vi "Transform And Project Single Object.vi"(6 "Backface Culling Enabled":bool, 7 "Light Direction":T1={"x"=0.0, "y"=10.0, "z"=-10.0}, 8 "Object":T3 {"Triangles"."Vertex 3"."UV"."v" min=0 max=1 step=0.1; "Triangles"."Vertex 3"."UV"."u" min=0 max=1 step=0.1; "Triangles"."Vertex 2"."UV"."v" min=0 max=1 step=0.1; "Triangles"."Vertex 2"."UV"."u" min=0 max=1 step=0.1; "Triangles"."Vertex 1"."UV"."v" min=0 max=1 step=0.1; "Triangles"."Vertex 1"."UV"."u" min=0 max=1 step=0.1}, 9 "View Matrix":sgl[][](array[numeric]), 10 "Projection Matrix":sgl[][](array[numeric]), 11 "Screen Dimensions":T2) -> (3 "Triangles":T4[](array[typedef]) {"Vertex 3"."UV"."v" min=0 max=1 step=0.1; "Vertex 3"."UV"."u" min=0 max=1 step=0.1; "Vertex 2"."UV"."v" min=0 max=1 step=0.1; "Vertex 2"."UV"."u" min=0 max=1 step=0.1; "Vertex 1"."UV"."v" min=0 max=1 step=0.1; "Vertex 1"."UV"."u" min=0 max=1 step=0.1})   [LabVIEW 2020, in "Scene.lvclass"]
uses:
  Scene/Scene.lvclass
  Scene/Scene.lvclass/Scene.ctl
  Graphics/Libraries/3D/3D.lvlib
  Graphics/Libraries/3D/Vector 3D.ctl
  Graphics/Libraries/Raster/UV.ctl
  Graphics/Libraries/Raster/Raster.lvlib
  Graphics/Libraries/3D/Vertex.ctl
  Graphics/Libraries/3D/Triangle.ctl
  Graphics/Libraries/Raster/Rectangle Dimensions.ctl
  Graphics/Libraries/Raster/Texture.ctl
  Graphics/Libraries/3D/Material.ctl
  Graphics/Libraries/3D/Transform.ctl
  Graphics/Libraries/3D/Object.ctl
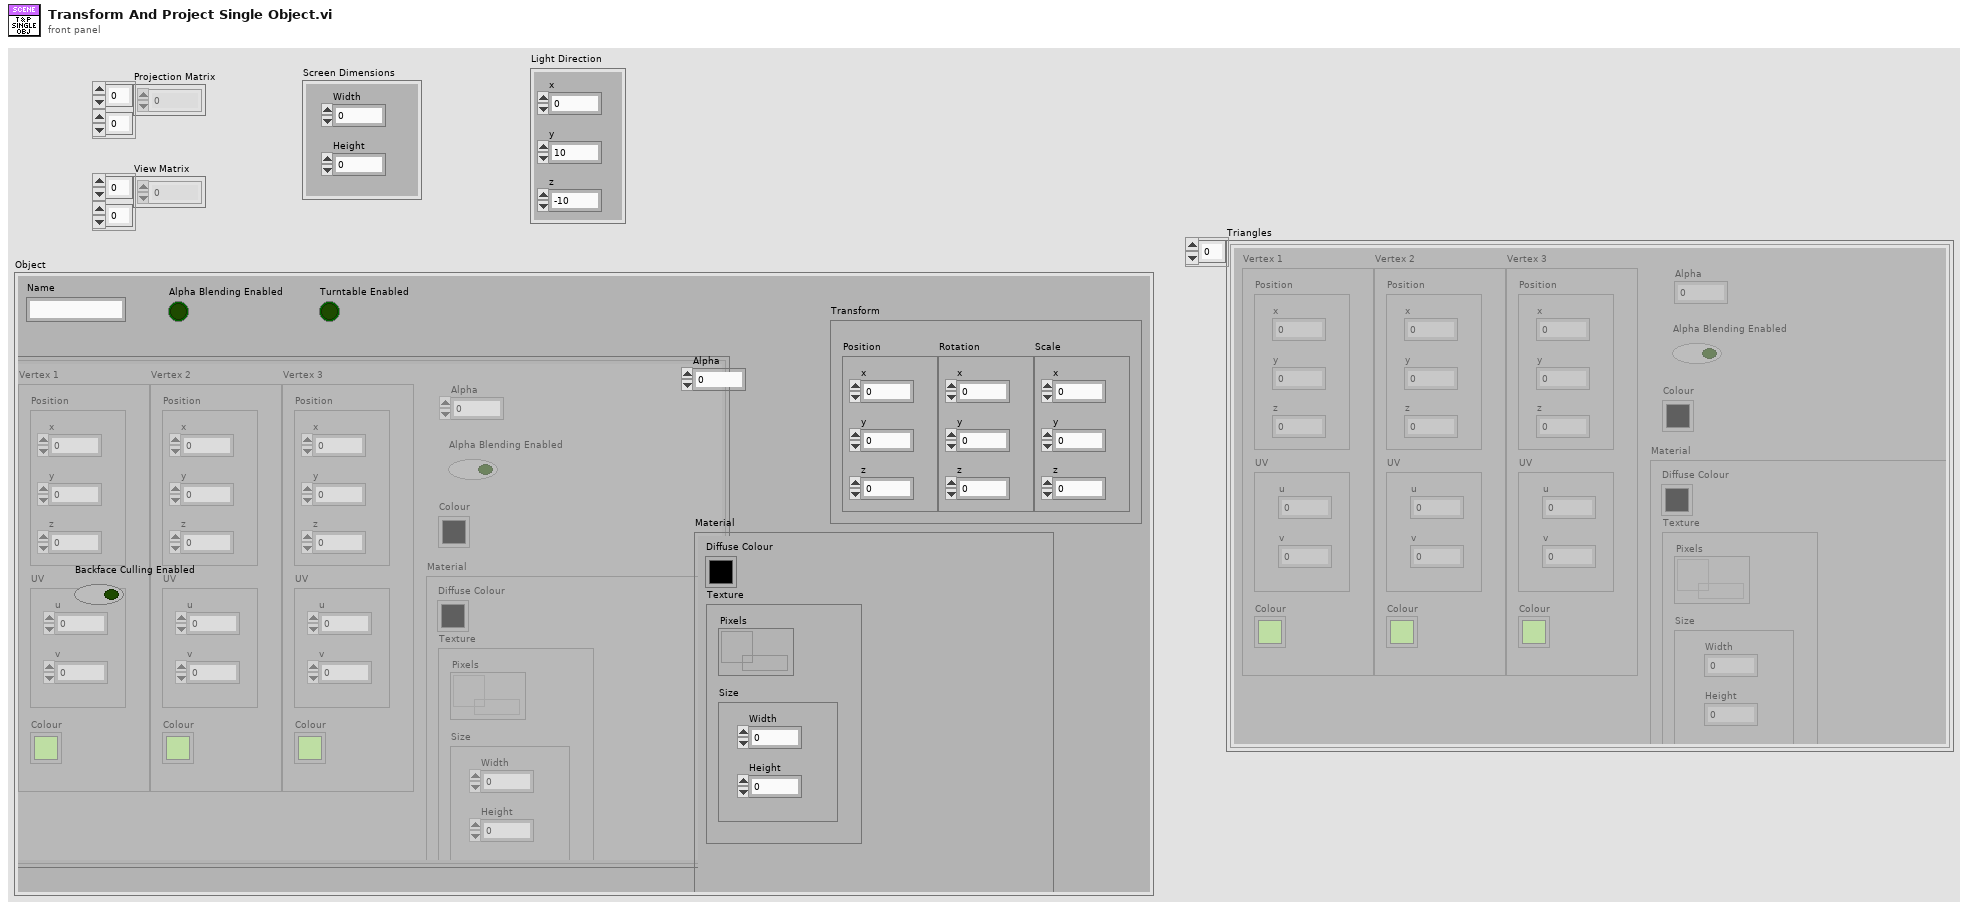
[diagram p1: front panel]
types:
  T1 = typedef "3D.lvlib/Vector 3D.ctl" = cluster{"x":sgl, "y":sgl, "z":sgl}
  T2 = typedef "Raster.lvlib/Rectangle Dimensions.ctl" = cluster{"Width":u32, "Height":u32}
  T3 = typedef "3D.lvlib/Object.ctl" = cluster{"Triangles":T4[], "Transform":T9, "Name":string, "Alpha Blending Enabled":bool, "Alpha":dbl, "Turntable Enabled":bool, "Material":T7}
  T4 = typedef "3D.lvlib/Triangle.ctl" = cluster{"Vertex 1":T5, "Vertex 2":T5, "Vertex 3":T5, "Alpha":dbl, "Alpha Blending Enabled":bool, "Colour":u32, "Material":T7}
  T5 = typedef "3D.lvlib/Vertex.ctl" = cluster{"Position":T1, "UV":T6, "Colour":u32}
  T6 = typedef "Raster.lvlib/UV.ctl" = cluster{"u":sgl, "v":sgl}
  T7 = typedef "3D.lvlib/Material.ctl" = cluster{"Diffuse Colour":u32, "Texture":T8}
  T8 = typedef "Raster.lvlib/Texture.ctl" = cluster{"Pixels":refnum<data-value>, "Size":T2}
  T9 = typedef "3D.lvlib/Transform.ctl" = cluster{"Position":T1, "Rotation":T1, "Scale":T1}
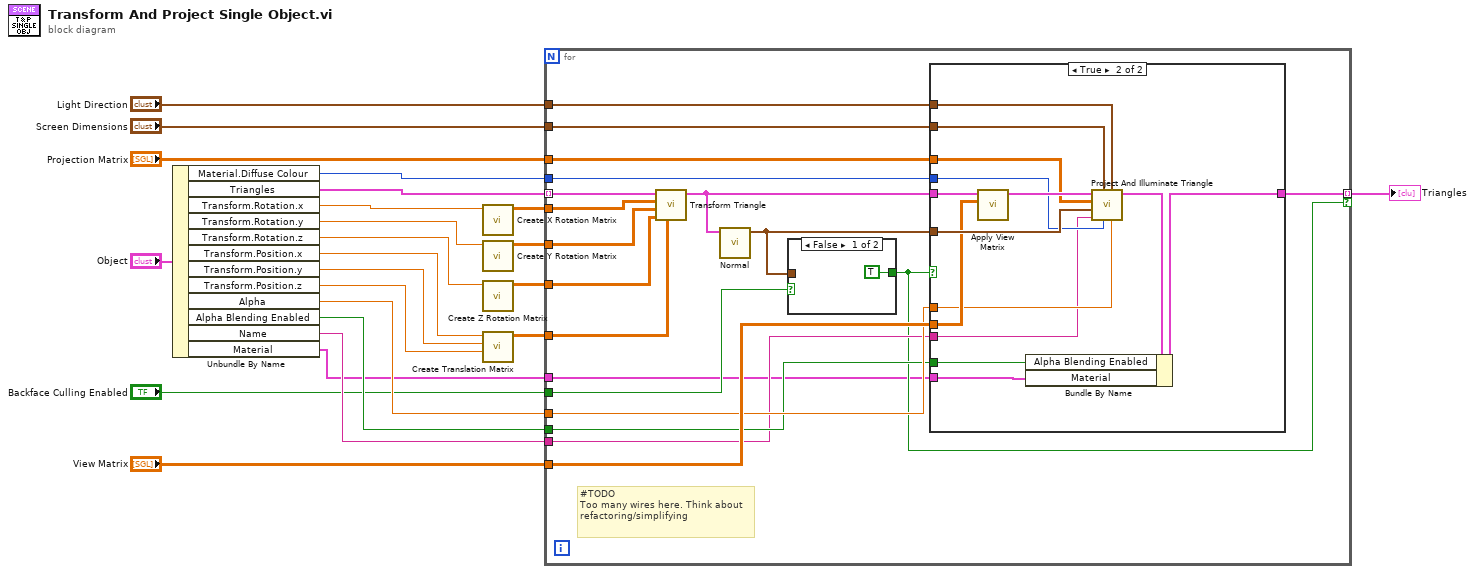
[diagram p0: block diagram]
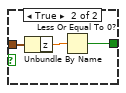
[diagram p2: hidden frame]
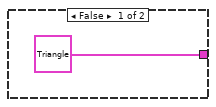
[diagram p3: hidden frame]
diagram:
  n1 = Unbundle By Name("Object") -> ("Material.Diffuse Colour"=w15:u32, "Triangles"=w8:T4[], "Transform.Rotation.x"=w16:sgl, "Transform.Rotation.y"=w17:sgl, "Transform.Rotation.z"=w18:sgl, "Transform.Position.x"=w19:sgl, "Transform.Position.y"=w20:sgl, "Transform.Position.z"=w21:sgl, "Alpha"=w22:dbl, "Alpha Blending Enabled"=w5:bool, "Name"=w3:string, "Material"=w1:T7)
  n2 = call "Create X Rotation Matrix.vi"("Theta (°)"=w16) -> ("Rotation X Matrix"=w11:sgl[][])  [unwired: 10 in]
  n3 = call "Create Y Rotation Matrix.vi"("Theta (°)"=w17) -> ("Rotation Y Matrix"=w10:sgl[][])  [unwired: 10 in]
  n4 = call "Create Z Rotation Matrix.vi"("Theta (°)"=w18) -> ("Rotation Z Matrix"=w12:sgl[][])  [unwired: 10 in]
  n5 = call "Create Translation Matrix.vi"("z"=w21, "y"=w20, "x"=w19) -> ("Translation Matrix"=w9:sgl[][])  [unwired: 8 in]
  n6 = for {
    tunnel: w12 -> [w38]
    tunnel: w11 -> [w40]
    tunnel: [w42] -> w23 mode=indexing if=w26
    tunnel: w10 -> [w39]
    tunnel: w9 -> [w37]
    tunnel: w8 -> [w34] mode=indexing
    tunnel: "View Matrix" -> [w36]
    tunnel: w15 -> [w33]
    tunnel: w22 -> [w32]
    tunnel: "Screen Dimensions" -> [w31]
    tunnel: "Projection Matrix" -> [w30]
    tunnel: w5 -> [w29]
    tunnel: "Light Direction" -> [w28]
    tunnel: w3 -> [w27]
    tunnel: "Backface Culling Enabled" -> [w25]
    tunnel: w1 -> [w24]
    # "#TODO\nToo many wires here. Think about refactoring/simplifying"
    n7 = call "Transform Triangle.vi"("Translation Matrix"=w37, "Rotation Z Matrix"=w38, "Rotation Y Matrix"=w39, "Rotation X Matrix"=w40, "Triangle in"=w34) -> ("Triangle out"=w35:T4)  [unwired: 6 in]
    n8 = call "Normal.vi"("Triangle"=w35) -> ("Normal"=w41:T1)  [unwired: 10 in]
    n9 = case shown="False" w25 {
      tunnel: w41 -> [_ w45]
      tunnel: [TRUE w44] -> w26
      frame False {
      }
      frame True {
        n10 = Unbundle By Name(w45) -> ("z"=w46:sgl)
        n11 = Less Or Equal To 0?(x=w46) -> (x <= 0?=w44:bool)
      }
    }
    n12 = case shown="True" w26 {
      tunnel: [T4 {"Vertex 1"={"Position"={"x"=0.0, "y"=0.0, "z"=0.0}, "UV"={"u"=0.0, "v"=0.0}, "Colour"=12517256}, "Vertex 2"={"Position"={"x"=0.0, "y"=0.0, "z"=0.0}, "UV"={"u"=0.0, "v"=0.0}, "Colour"=12517256}, "Vertex 3"={"Position"={"x"=0.0, "y"=0.0, "z"=0.0}, "UV"={"u"=0.0, "v"=0.0}, "Colour"=12517256}, "Alpha"=12517256.0, "Alpha Blending Enabled"=FALSE, "Colour"=0, "Material"={"Diffuse Colour"=0, "Texture"={"Pixels"=refnum, "Size"={"Width"=0, "Height"=0}}}} ("Cluster") w52] -> w42
      tunnel: w41 -> [_ w61]
      tunnel: w35 -> [_ w59]
      tunnel: w36 -> [_ w58]
      tunnel: w33 -> [_ w57]
      tunnel: w32 -> [_ w56]
      tunnel: w31 -> [_ w55]
      tunnel: w30 -> [_ w54]
      tunnel: w29 -> [_ w51]
      tunnel: w28 -> [_ w50]
      tunnel: w27 -> [_ w49]
      tunnel: w24 -> [_ w48]
      frame False {
      }
      frame True {
        n13 = call "Apply View Matrix.vi"("View Matrix"=w58, "Triangle in"=w59) -> ("Triangle out"=w60:T4)  [unwired: 9 in]
        n14 = call "Project And Illuminate Triangle.vi"("Alpha"=w56, "Light Direction"=w50, "Diffuse Colour"=w57, "Screen Dimensions"=w55, "Name"=w49, "Normal"=w61, "Projection Matrix"=w54, "Triangle in"=w60) -> ("Triangle out"=w53:T4)  [unwired: 3 in]
        n15 = Bundle By Name(cluster=w53, "Alpha Blending Enabled"=w51, "Material"=w48) -> (w52:T4)
      }
    }
  }
  "Triangles" <- w23
